vi "Peak.vi"(11 "TypedCircularBuffer in":refnum<class "VarCircularBuffer.lvclass">) -> (2 "element":variant=variant(i32 0), 3 "TypedCircularBuffer out":refnum<class "VarCircularBuffer.lvclass">)   [LabVIEW 2024, in "VarCircularBuffer.lvclass"]
uses:
  VarCircularBuffer.lvclass
  VarCircularBuffer.lvclass/VarCircularBuffer.ctl
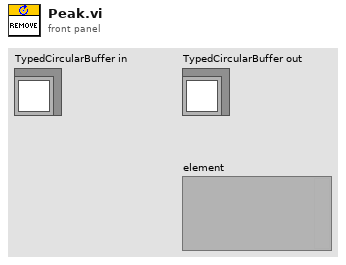
[diagram p1: front panel]
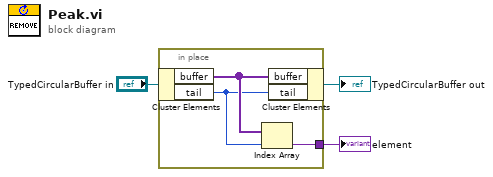
[diagram p0: block diagram]
diagram:
  n1 = in-place {
    in-place-border: [w5] -> w1
    n2 = in-place-cluster #1("TypedCircularBuffer in") -> ("buffer"=w6:variant[], "tail"=w4:u32)
    n3 = Index Array(array=w6, index=w4) -> (element=w5:variant)
    n4 = in-place-cluster #1("buffer"=w6, "tail"=w4) -> (→"TypedCircularBuffer out":refnum<class "VarCircularBuffer.lvclass">)
  }
  "element" <- w1
